vi "2015 Check Summary Header.vi"(8 "Error In":errorcluster, 11 "Summary File":path) -> (0 "Error Out":errorcluster, 2 "Write Header?":bool, 3 "Summary Path":path)   [LabVIEW 2014]
uses:
  <vilib>/Utility/file.llb/Read From Spreadsheet File (string).vi
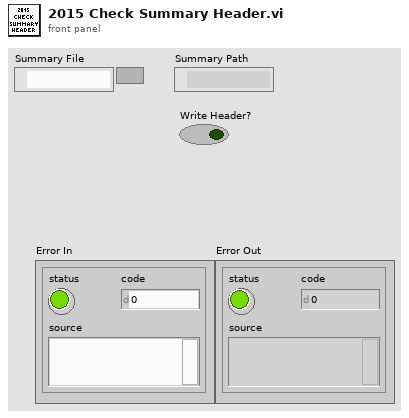
[diagram p1: front panel]
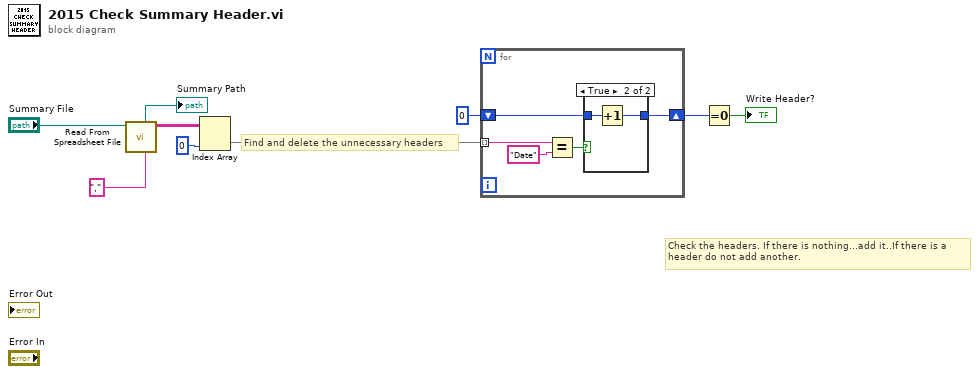
[diagram p0: block diagram]
diagram:
  # "Find and delete the unnecessary headers"
  # "Check the headers. If there is nothing...add it..If there is a \nheader do not add another."
  n1 = call-poly <vilib>:"Read From Spreadsheet File.vi"("delimiter (\\t)"="," ("delimiter (\\t)"), "file path (dialog if empty)"="Summary File") -> ("all rows"=w3:string[][], "new file path (Not A Path if cancelled)"=→"Summary Path":path)  [unwired: 5 in, 3 out]
  n2 = Index Array(array=w3, index (col)=0 ("disabled index (col)")) -> (element=w5:string[])  [unwired: 1 in]
  n3 = for {
    tunnel: w5 -> [w14] mode=indexing
    shift-right: [w10] -> w8
    shift-left: 0 -> [w11]
    n4 = Equal?(x=w14, y="Date") -> (x = y?=w12:bool)
    n5 = case shown="True" w12 {
      tunnel: w11 -> [w15 w17]
      tunnel: [w15 w16] -> w10
      frame False {
      }
      frame True {
        n6 = Increment(x=w17) -> (x+1=w16:i32)
      }
    }
  }
  n7 = Equal To 0?(x=w8) -> (x = 0?=→"Write Header?":bool)
